vi "Drive Controller.vi"(8 "error in":errorcluster) -> ()   [LabVIEW 2015]
doc: "This VI executes continuously carrying out the current operation and responding to updates or new operation requests. It will often contain the timing or control code that is difficult to place directly in TeleOp. This VI generally opens all sensors and motors and isolates the rest of the robot code from knowing implementation details of how the operations are carried out."
uses:
  <vilib>/Rock Robotics/WPI/CAN/TalonSRX/WPI_CANTalonSRX_GlobalStatus.ctl
  Drive Setpoints.ctl
  Drive Operations.ctl
  <vilib>/Rock Robotics/WPI/SafetyOutput/WPI_SafetyOutputConfigMenu.ctl
  <vilib>/Rock Robotics/WPI/CAN/TalonSRX/WPI_CANTalonSRX_APIControlMode.ctl
  JoystickData.ctl
  <vilib>/Rock Robotics/WPI/MotorControl/WPI_MotorControlOpenCANTalonSRX.vi
  <vilib>/Rock Robotics/WPI/Utilities/WPI_GetSetVariantRefNum.vi
  Global Drive Variables.vi
  NavX/NavX Global.vi
  <vilib>/Rock Robotics/WPI/Joystick/WPI_JoystickArcadeMapping.vi
  LED Lights/LED Lights Global.vi
panel:
  out "Speed":dbl
  out "Angle To Turn":dbl
  out "Talon SRX Status 2":T1
  out "Talon SRX Status":T1
  out "Setpoints":T2(graph)
  out "Current\nCmd":string
  # "Tip: It may be helpful to observe inputs and sensor values.\nYou may also want to display tuning or debugging controls."
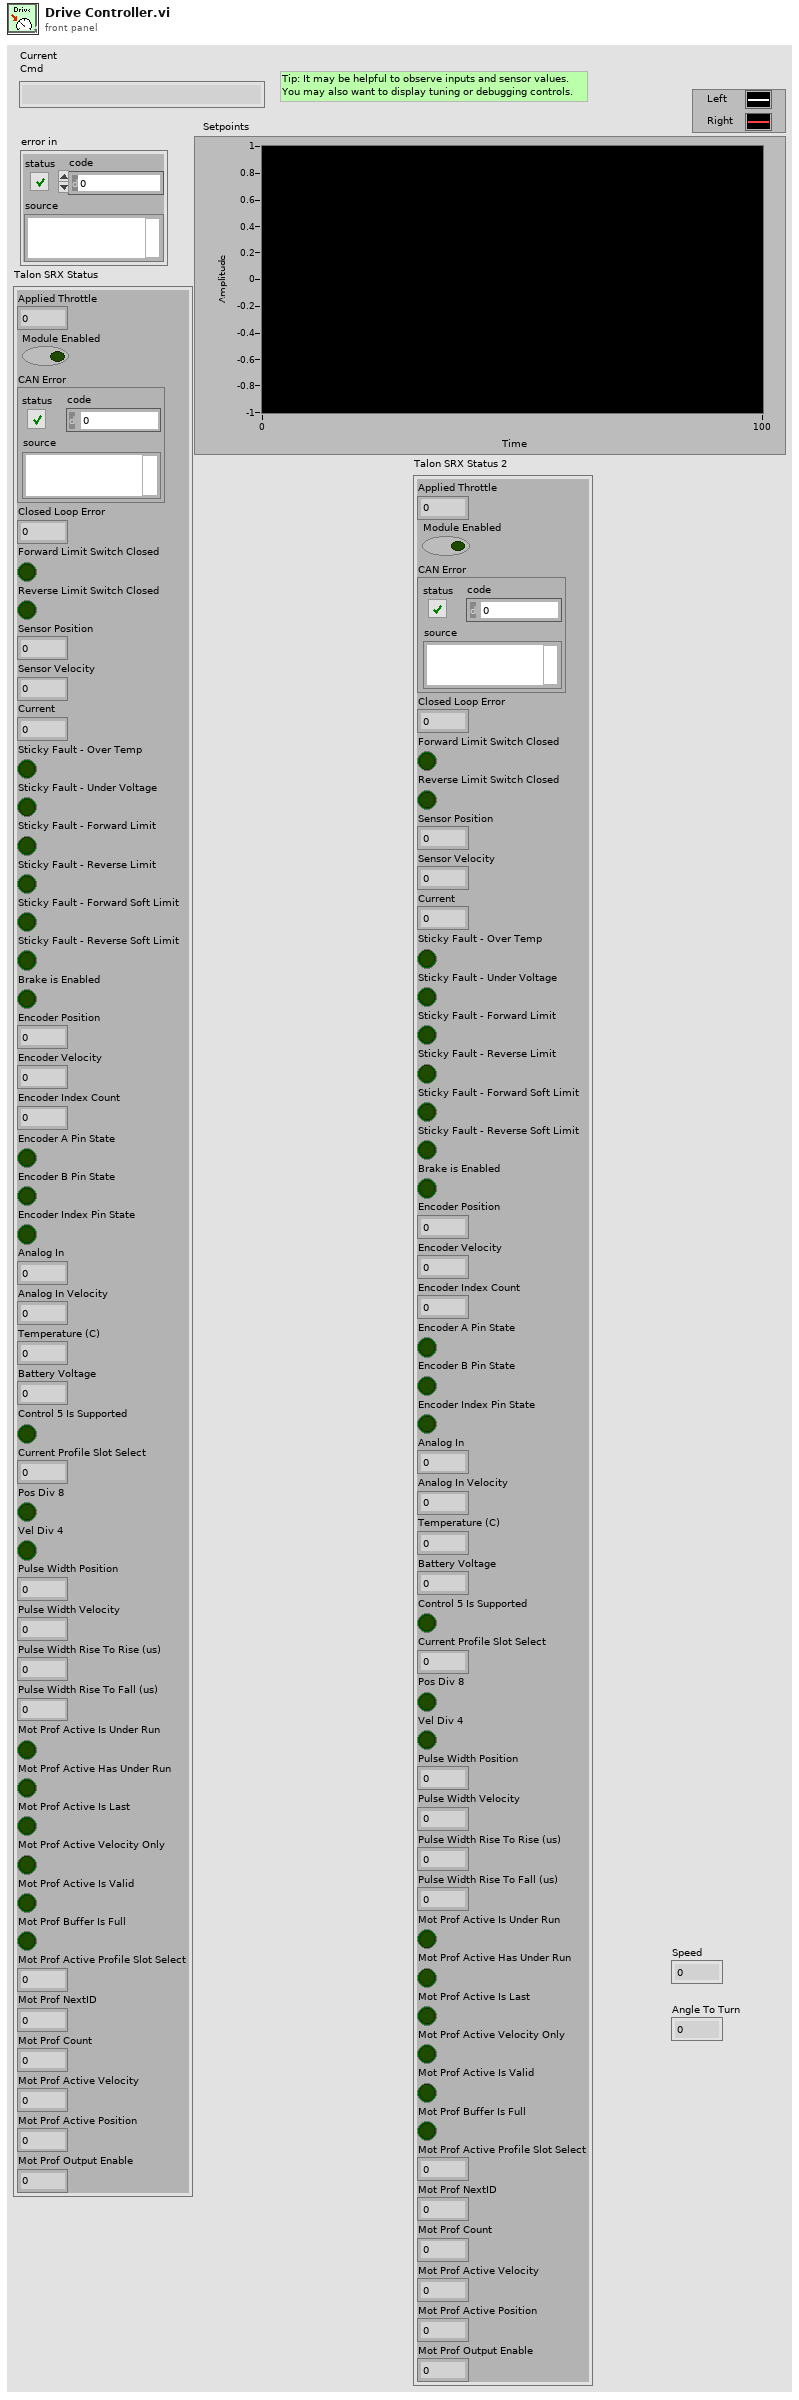
[diagram p1: front panel]
types:
  T1 = typedef "WPI_CANTalonSRX_GlobalStatus.ctl" = cluster{"Applied Throttle":dbl, "Module Enabled":bool, "CAN Error":errorcluster, "Closed Loop Error":dbl, "Forward Limit Switch Closed":bool, "Reverse Limit Switch Closed":bool, "Sensor Position":dbl, "Sensor Velocity":dbl, "Current":dbl, "Sticky Fault - Over Temp":bool, "Sticky Fault - Under Voltage":bool, "Sticky Fault - Forward Limit":bool, "Sticky Fault - Reverse Limit":bool, "Sticky Fault - Forward Soft Limit":bool, "Sticky Fault - Reverse Soft Limit":bool, "Brake is Enabled":bool, "Encoder Position":dbl, "Encoder Velocity":dbl, "Encoder Index Count":dbl, "Encoder A Pin State":bool, "Encoder B Pin State":bool, "Encoder Index Pin State":bool, "Analog In":dbl, "Analog In Velocity":dbl, "Temperature (C)":dbl, "Battery Voltage":dbl, "Control 5 Is Supported":bool, "Current Profile Slot Select":dbl, "Pos Div 8":bool, "Vel Div 4":bool, "Pulse Width Position":i32, "Pulse Width Velocity":i32, "Pulse Width Rise To Rise (us)":i32, "Pulse Width Rise To Fall (us)":i32, "Mot Prof Active Is Under Run":bool, "Mot Prof Active Has Under Run":bool, "Mot Prof Active Is Last":bool, "Mot Prof Active Velocity Only":bool, "Mot Prof Active Is Valid":bool, "Mot Prof Buffer Is Full":bool, "Mot Prof Active Profile Slot Select":i32, "Mot Prof NextID":i32, "Mot Prof Count":i32, "Mot Prof Active Velocity":dbl, "Mot Prof Active Position":dbl, "Mot Prof Output Enable":i32}
  T2 = cluster{"Left Setpoint":dbl, "Right Setpoint":dbl}
  T3 = typedef "WPI_CANTalonSRX_APIControlMode.ctl" = enum8{"Percent VBus", "Speed", "Position", "Slave", "Unchanged / Invalid", "Voltage Compensation", "Current", "Motion Profile"}
  T4 = typedef "WPI_SafetyOutputConfigMenu.ctl" = enum16{"Enable", "Disable"}
  T5 = typedef "Drive Setpoints.ctl" = cluster{"Operation":T6, "Left Setpoint":dbl, "Right Setpoint":dbl, "Duration":dbl, "Angle":dbl}
  T6 = typedef "Drive Operations.ctl" = enum16{"Reserve", "Read Current", "Immediate", "Drive for Time", "Drive for Distance", "Turn Degrees"}
  T7 = typedef "Drive Global Type Def.ctl" = cluster{"Left Drive Motors":cluster{"Motor Front":T8, "Motor Back":T8, "Motor Errors":errorcluster}, "Right Drive Motors":cluster{"Motor Front":T8, "Motor Back":T8, "Motor Errors":errorcluster}}
  T8 = typedef "Motor Global Type Def.ctl" = cluster{"Motor Error":errorcluster}
  T9 = typedef "WPI_MotorControlDeviceRef.ctl" = cluster{"DeviceStatus":errorcluster, "Type":T10, "PWM":cluster{"PWM Channel":T11, "DeadBand":T12}, "CAN":cluster{"Device Number":u8, "Control Mode":T13, "Semaphore":T14, "Max Vout":dbl, "TalonSRX Control Mode":T3}, "Invert":bool}
  T10 = typedef "WPI_MotorControlType.ctl" = enum16{"PWM", "CAN", "CANTalonSRX"}
  T11 = typedef "FPGA_DIOPWMChannel.ctl" = enum8{"PWM 0", "PWM 1", "PWM 2", "PWM 3", "PWM 4", "PWM 5", "PWM 6", "PWM 7", "PWM 8", "PWM 9", "PWM MXP 0", "PWM MXP 1", "PWM MXP 2", "PWM MXP 3", "PWM MXP 4", "PWM MXP 5", "PWM MXP 6", "PWM MXP 7", "PWM MXP 8", "PWM MXP 9", "Invalid"}
  T12 = typedef "WPI_PWMDeadband.ctl" = cluster{"Name":string, "maxPositivePwm":i32, "minPositivePwm":i32, "centerPwm":i32, "maxNegativePwm":i32, "minNegativePwm":i32, "angularRange":u16}
  T13 = typedef "WPI_CANJaguar_ControlMode.ctl" = enum8{"Percent VBus", "Current", "Speed", "Position", "Voltage"}
  T14 = typedef "Semaphore RefNum" = refnum<k1>
  T15 = typedef "WPI_RobotDriveDevRef.ctl" = cluster{"DevStatus":errorcluster, "Motors[]":T9[], "Square Inputs":bool, "Max Output":dbl}
  T16 = typedef "Command Status Info.ctl" = cluster{"Name":string, "Status":T17, "notifier out":T18}
  T17 = typedef "Completion Status.ctl" = enum16{"Successful", "Aborted", "Incomplete"}
  T18 = typedef "Completion Notifier.ctl" = refnum<notifier>
  T19 = cluster{"SubSystem Data":T5, cluster{"Start Time (ms)":u32, "Iterations":i32}, cluster{"Command Info":T16, "Description":string, "SubSystem Data":T5, "notifier out":refnum<notifier>, "Subsystem Name":string}}
  T20 = typedef "navX-MXP IMU.lvlib/navX YPRH Data.ctl" = cluster{"Yaw":dbl, "Pitch":dbl, "Roll":dbl, "Heading":dbl}
  T21 = cluster{"SubSystem Data":T5, cluster{"Start Time (ms)":u32, "Iterations":i32}, "Default Command Arguments":cluster{"Command Info":T16, "Description":string, "SubSystem Data":T5, "notifier out":refnum<notifier>, "Subsystem Name":string}}
  T22 = cluster{"Left Motor Value":dbl, "Right Motor Value":dbl}
  T23 = typedef "JoystickData.ctl" = cluster{"Axes":dbl[], "Buttons":bool[]}
  T24 = typedef "WPI_JoystickDevRef.ctl" = cluster{"Device":T25}
  T25 = typedef "WPI_JoystickDeviceEnum.ctl" = enum16{"USB 0", "USB 1", "USB 2", "USB 3", "USB 4", "USB 5"}
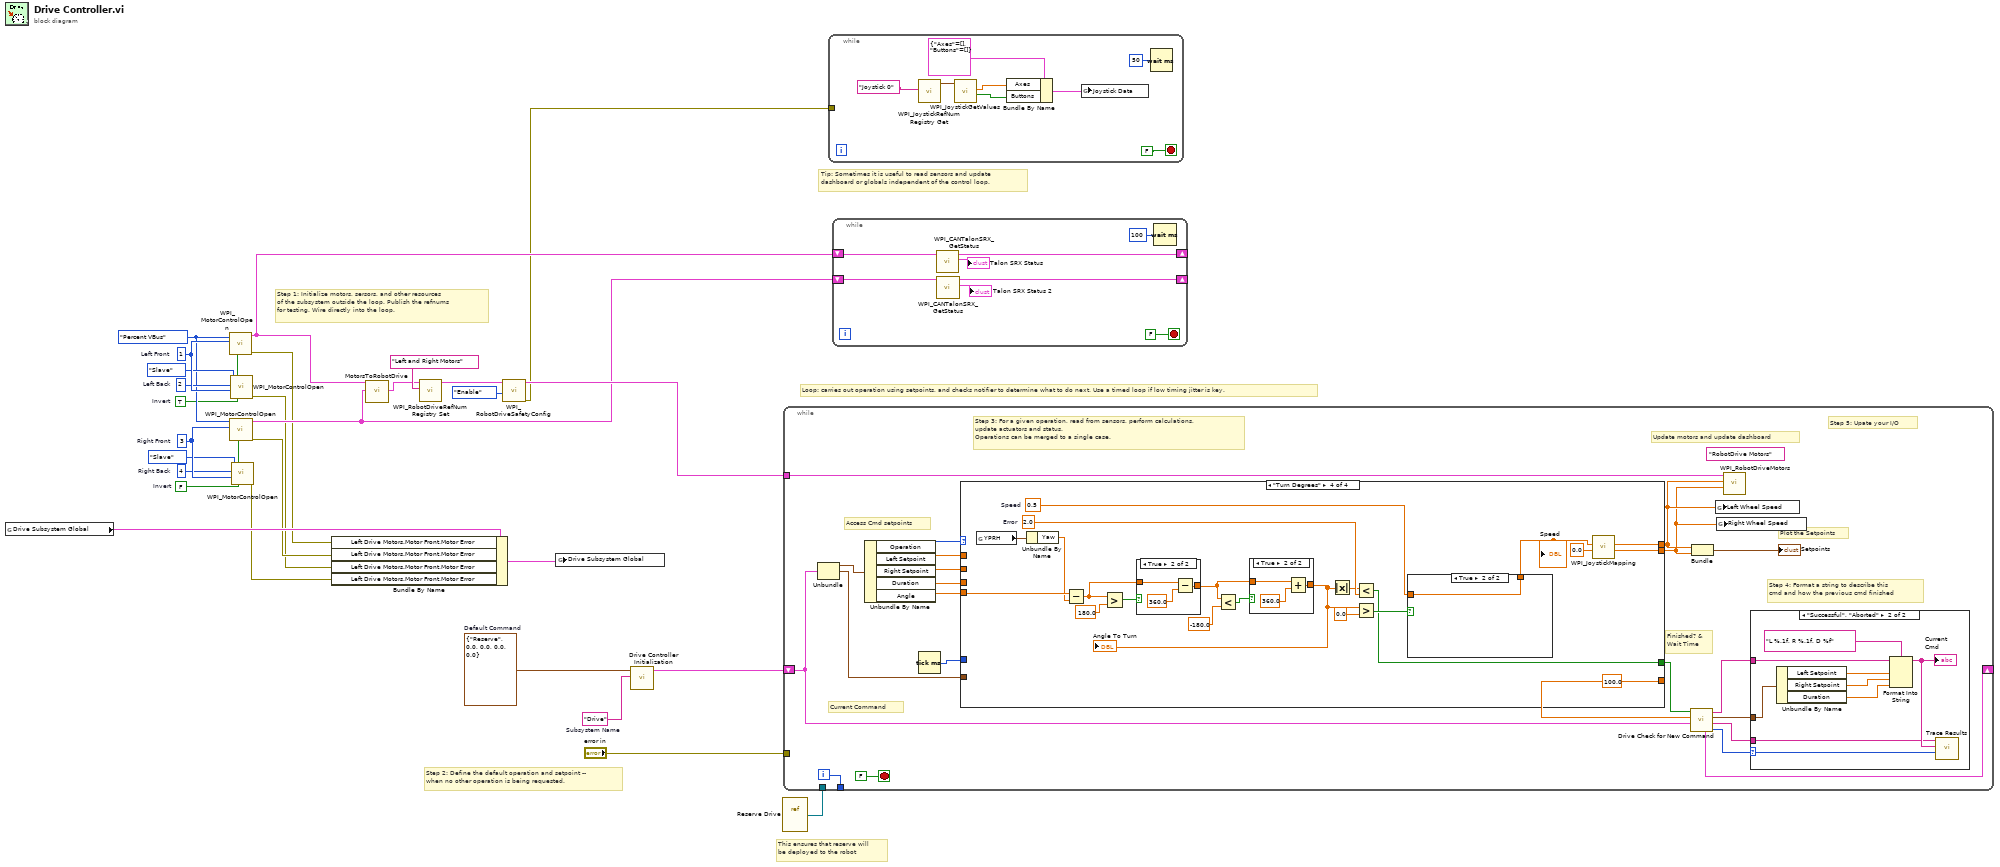
[diagram p0: block diagram]
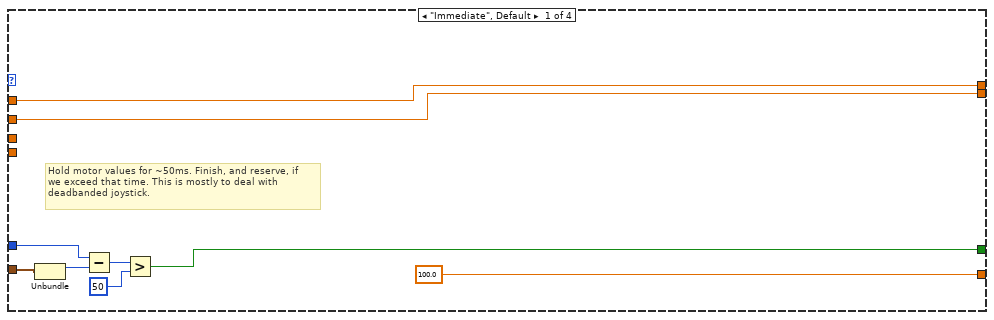
[diagram p3: hidden frame]
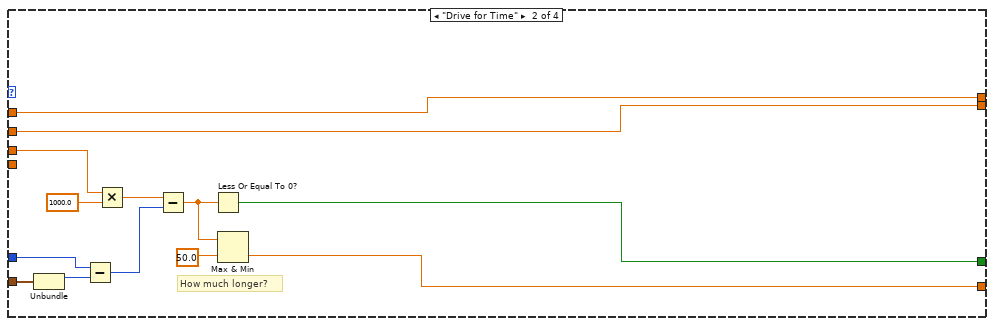
[diagram p4: hidden frame]
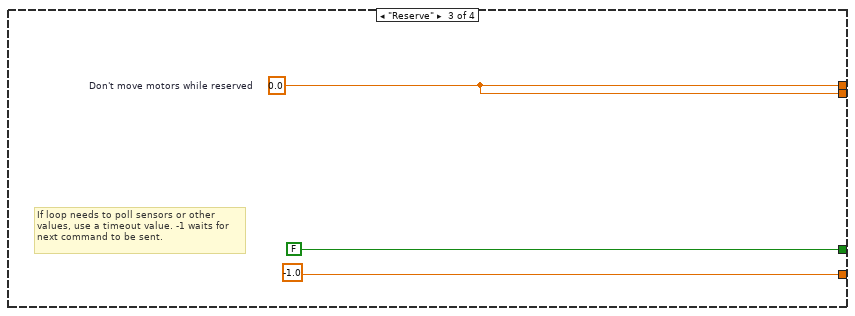
[diagram p5: hidden frame]
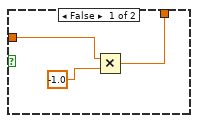
[diagram p8: hidden frame]
diagram:
  w8 = TRUE  # Invert
  w9 = FALSE  # Invert
  w14 = u8 4  # Right Back
  w15 = u8 3  # Right Front
  w17 = u8 2  # Left Back
  w18 = u8 1  # Left Front
  w12 = WPI_CANTalonSRX_APIControlMode."Percent VBus" ("Control Mode")
  w27 = T5 {"Operation"=enum."Reserve", "Left Setpoint"=0.0, "Right Setpoint"=0.0, "Duration"=0.0, "Angle"=0.0}  # Default Command
  w28 = "Drive"  # Subsystem Name
  # "This ensures that reserve will\nbe deployed to the robot"
  # "Tip: Sometimes it is useful to read sensors and update\ndashboard or globals independent of the control loop."
  # "Step 2: Define the default operation and setpoint --\nwhen no other operation is being requested."
  # "Step 1: Initialize motors, sersors, and other resources\nof the subsystem outside the loop. Publish the refnums\nfor testing. Wire directly into the loop."
  # "Loop: carries out operation using setpoints, and checks notifier to determine what to do next. Use a timed loop if low timing jitter is key."
  n1 = global read "LED Lights Global.vi" "Drive Subsystem Global"() -> (w6:T7)
  n2 = call-poly <vilib>:"WPI_MotorControlOpen.vi"("Invert"=w8, "Device Number"=w18, "Control Mode"=w12) -> ("error out"=w5:errorcluster, "MotorControlDeviceRef"=w11:T9)  [unwired: 7 in]
  n3 = call-poly <vilib>:"WPI_MotorControlOpen.vi"("Invert"=w9, "Device Number"=w15, "Control Mode"=w12) -> ("error out"=w4:errorcluster, "MotorControlDeviceRef"=w10:T9)  [unwired: 7 in]
  n4 = call-poly <vilib>:"WPI_MotorControlOpen.vi"("Master Device Number"=w18, "Device Number"=w17, "Control Mode"=WPI_CANTalonSRX_APIControlMode."Slave") -> ("error out"=w3:errorcluster)  [unwired: 7 in, 1 out]
  n5 = call-poly <vilib>:"WPI_MotorControlOpen.vi"("Master Device Number"=w15, "Device Number"=w14, "Control Mode"=WPI_CANTalonSRX_APIControlMode."Slave") -> ("error out"=w2:errorcluster)  [unwired: 7 in, 1 out]
  n6 = Bundle By Name(cluster=w6, "Left Drive Motors.Motor Front.Motor Error"=w5, "Left Drive Motors.Motor Front.Motor Error"=w4, "Left Drive Motors.Motor Front.Motor Error"=w3, "Left Drive Motors.Motor Front.Motor Error"=w2) -> (w1:T7)
  n7 = call "MotorsToRobotDrive.vi"("Left"=w11, "Right"=w10) -> ("RobotDriveDevRef"=w19:T15)  [unwired: 16 in, 1 out]
  n8 = call <vilib>:"WPI_RobotDriveRefNum Registry Set.vi"("refnum name"="Left and Right Motors", "RobotDriveDevRef"=w19) -> ("RobotDriveDevRef"=w25:T15)  [unwired: 2 in, 7 out]
  n9 = call <vilib>:"WPI_RobotDriveSafetyConfig.vi"("mode"=WPI_SafetyOutputConfigMenu."Enable", "RobotDriveDevRef"=w25) -> ("error out"=w7:errorcluster, "RobotDriveDevRef"=w23:T15)  [unwired: 8 in]
  n10 = global write "LED Lights Global.vi" "Drive Subsystem Global"(w1) -> ()
  n11 = call "Drive Controller Initialization.vi"("Subsystem Name"=w28, "Default Command"=w27) -> ("output cluster"=w21:T19)  [unwired: 9 in]
  n12 = vi-ref "Reserve Drive.vi"() -> (w20:refnum<vi>)
  n13 = while {
    shift-right: [w39] -> _
    shift-left: w21 -> [w32]
    tunnel: [w49] -> _
    tunnel: w23 -> [w47]
    tunnel: "error in" -> [_]
    tunnel: w20 -> [_]
    i -> [w49]
    stop <- FALSE stop-if-true
    (unwired) "RobotDrive Motors" ("Name")
    # "Step 5: Upate your I/O"
    # "Step 4: Format a string to describe this\ncmd and how the previous cmd finished"
    # "Current Command"
    # "Update motors and update dashboard"
    # "Plot the Setpoints"
    # "Access Cmd setpoints"
    # "Finished? &\nWait Time"
    # "Step 3: For a given operation, read from sensors, perform calculations,\nupdate actuators and status.\nOperations can be merged to a single case."
    n14 = Unbundle(w32) -> ("SubSystem Data"=w46:T5, w33:cluster{"Start Time (ms)":u32, "Iterations":i32})  [unwired: 1 out]
    n15 = Unbundle By Name(w46) -> ("Operation"=w45:T6, "Left Setpoint"=w44:dbl, "Right Setpoint"=w43:dbl, "Duration"=w42:dbl, "Angle"=w29:dbl)
    n16 = Tick Count (ms)() -> (millisecond timer value=w41:u32)
    n17 = case shown="\"Turn Degrees\"" w45 {
      tunnel: [100.0 w69 -1.0 100.0] -> w38
      tunnel: [w61 w76 FALSE ("ignore previous (F)") w87] -> w37
      tunnel: w33 -> [w60 w78 _ _]
      tunnel: [w67 w75 w82 w104] -> w31
      tunnel: [w66 w74 w82 w103] -> w30
      tunnel: w44 -> [w67 w75 _ _]
      tunnel: w43 -> [w66 w74 _ _]
      tunnel: w42 -> [_ w73 _ _]
      tunnel: w41 -> [w62 w72 _ _]
      tunnel: w29 -> [_ _ _ w101]
      frame "Immediate", Default {
        # "Hold motor values for ~50ms. Finish, and reserve, if\nwe exceed that time. This is mostly to deal with\ndeadbanded joystick."
        n18 = Unbundle(w60) -> ("Start Time (ms)"=w63:u32)  [unwired: 1 out]
        n19 = Subtract(x=w62, y=w63) -> (x-y=w64:u32)
        n20 = Greater?(x=w64, y=u8 50 ("Left Motor")) -> (0:w61:bool)
      }
      frame "Drive for Time" {
        # "How much longer?"
        n21 = Unbundle(w78) -> ("Start Time (ms)"=w77:u32)  [unwired: 1 out]
        n22 = Subtract(x=w72, y=w77) -> (x-y=w81:u32)
        n23 = Multiply(x=w73, y=1000.0) -> (x*y=w80:dbl)
        n24 = Subtract(x=w80, y=w81) -> (x-y=w71:dbl)
        n25 = Less Or Equal To 0?(x=w71) -> (x <= 0?=w76:bool)
        n26 = Max & Min(x=w71, y=50.0) -> (min(x,y)=w69:dbl)  [unwired: 1 out]
      }
      frame "Reserve" {
        w82 = 0.0  # Don't move motors while reserved
        # "If loop needs to poll sensors or other\nvalues, use a timeout value. -1 waits for\nnext command to be sent."
      }
      frame "Turn Degrees" {
        w88 = 2.0  # Error
        w95 = 0.5  # Speed
        n27 = global read "NavX Global.vi" "YPRH"() -> (w100:T20)
        n28 = Unbundle By Name(w100) -> ("Yaw"=w99:dbl)
        n29 = Subtract(x=w101, y=w99) -> (x-y=w92:dbl)
        n30 = Greater?(x=w92, y=180.0) -> (0:w93:bool)
        n31 = case shown="True" w93 {
          tunnel: w92 -> [w110 w113]
          tunnel: [w110 w111] -> w89
          frame False {
          }
          frame True {
            n32 = Subtract(x=w113, y=360.0) -> (x-y=w111:dbl)
          }
        }
        n33 = Less?(x=w89, y=-180.0) -> (x < y?=w90:bool)
        n34 = case shown="True" w90 {
          tunnel: w89 -> [w106 w109]
          tunnel: [w106 w107] -> w85
          frame False {
          }
          frame True {
            n35 = Add(x=w109, y=360.0) -> (x+y=w107:dbl)
          }
        }
        "Angle To Turn" <- w85
        n36 = Absolute Value(x=w85) -> (abs(x)=w86:dbl)
        n37 = Less?(x=w86, y=w88) -> (x < y?=w87:bool)
        n38 = Greater?(x=w85, y=0.0) -> (0:w97:bool)
        n39 = case shown="True" w97 {
          tunnel: [w114 w117] -> w96
          tunnel: w95 -> [w115 w117]
          frame False {
            n40 = Multiply(x=w115, y=-1.0) -> (x*y=w114:dbl)
          }
          frame True {
          }
        }
        "Speed" <- w96
        n41 = call-poly <vilib>:"WPI_JoystickMapping.vi"("Y axis value"=0.0, "X axis value"=w96) -> ("Right Motor Value"=w103:dbl, "Left Motor Value"=w104:dbl)  [unwired: 8 in]
      }
    }
    n42 = call "Drive Check for New Command.vi"("input cluster"=w32, "Wait time (ms)"=w38, "Finished?"=w37) -> ("Completion"=w40:T17, "Subsystem Name"=w34:string, "SetPoint"=w35:T5, "Initial Trace String"=w36:string, "output cluster"=w39:T21)  [unwired: 4 in]
    n43 = Bundle("Left Motor Value"=w31, "Right Motor Value"=w30) -> (→"Setpoints":T22)  [unwired: 1 in]
    n44 = global write "Global Drive Variables.vi" "Left Wheel Speed"(w31) -> ()
    n45 = global write "Global Drive Variables.vi" "Right Wheel Speed"(w30) -> ()
    n46 = call <vilib>:"WPI_RobotDriveMotors.vi"("RightSpeed"=w30, "LeftSpeed"=w31, "RobotDriveDevRef"=w47) -> ()  [unwired: 1 in, 8 out]
    n47 = case shown="\"Successful\", \"Aborted\"" w40 {
      selector: w40 -> [_ w59]
      tunnel: w36 -> [_ w54]
      tunnel: w35 -> [_ w55]
      tunnel: w34 -> [_ w51]
      frame "Incomplete", Default {
        # "Continuing current command"
      }
      frame "Successful", "Aborted" {
        # "Report and setup for next command"
        n48 = Unbundle By Name(w55) -> ("Left Setpoint"=w57:dbl, "Right Setpoint"=w58:dbl, "Duration"=w52:dbl)
        n49 = Format Into String(format string="L %.1f, R %.1f, D %f", initial string=w54, w57, w58, w52) -> (resulting string=w53:string)  [unwired: 1 in, 1 out]
        "Current\nCmd" <- w53
        n50 = call <vilib>:"Trace Results.vi"("Status of previous command"=w59, "Description"=w53, "Subsystem"=w51) -> ()  [unwired: 9 in]
      }
    }
  }
  n51 = while {
    tunnel: w7 -> [_]
    stop <- FALSE stop-if-true
    n52 = call <vilib>:"WPI_JoystickRefNum Registry Get.vi"("refnum name"="Joystick 0") -> ("JoystickDevRef"=w123:T24)  [unwired: 1 in, 9 out]
    n53 = call <vilib>:"WPI_JoystickGetValues.vi"("JoystickDevRef"=w123) -> ("Buttons"=w119:bool[], "Axes"=w120:dbl[])  [unwired: 6 in, 3 out]
    n54 = Bundle By Name(cluster=T23 {"Axes"=[], "Buttons"=[]} ("Joystick Data"), "Axes"=w120, "Buttons"=w119) -> (w118:T23)
    n55 = global write "Global Drive Variables.vi" "Joystick Data"(w118) -> ()
    n56 = Wait (ms)(milliseconds to wait=u32 50) -> ()  [unwired: 1 out]
  }
  n57 = while {
    shift-right: [w130] -> _
    shift-left: w11 -> [w131]
    shift-right: [w127] -> _
    shift-left: w10 -> [w128]
    stop <- FALSE stop-if-true
    n58 = call <vilib>:"WPI_CANTalonSRX_GetStatus.vi"("CAN Talon SRX Ref"=w131) -> ("Talon SRX Status"=→"Talon SRX Status":T1, "CAN Talon SRX Ref"=w130:T9)  [unwired: 8 in, 1 out]
    n59 = call <vilib>:"WPI_CANTalonSRX_GetStatus.vi"("CAN Talon SRX Ref"=w128) -> ("Talon SRX Status"=→"Talon SRX Status 2":T1, "CAN Talon SRX Ref"=w127:T9)  [unwired: 8 in, 1 out]
    n60 = Wait (ms)(milliseconds to wait=u32 100) -> ()  [unwired: 1 out]
  }
